vi "string.vi"() -> ()   [LabVIEW 2020]
panel:
  out "length":i32
  out "output":string
  in  "input":string
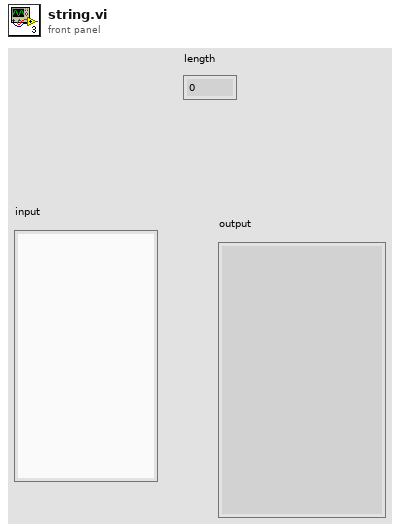
[diagram p1: front panel]
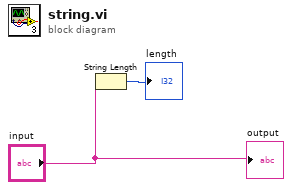
[diagram p0: block diagram]
diagram:
  n1 = String Length(string="input") -> (length=→"length":i32)
  "output" <- "input"
